vi "Reset.vi"(8 "error in (no error)":errorcluster, 10 "Reset":bool, 11 "ControlState in":T1 {"ChainMask" format="0x%02x"}) -> (0 "error out":errorcluster, 3 "ControlState out":T1 {"ChainMask" format="0x%02x"})   [LabVIEW 2018, in "ArduinoSerialBling.lvlib"]
uses:
  ArduinoSerialBling.lvlib
  ControlState.ctl
  ConnectionType.ctl
  UdpConnection.ctl
  ChainState.ctl
  TransmissionType.ctl
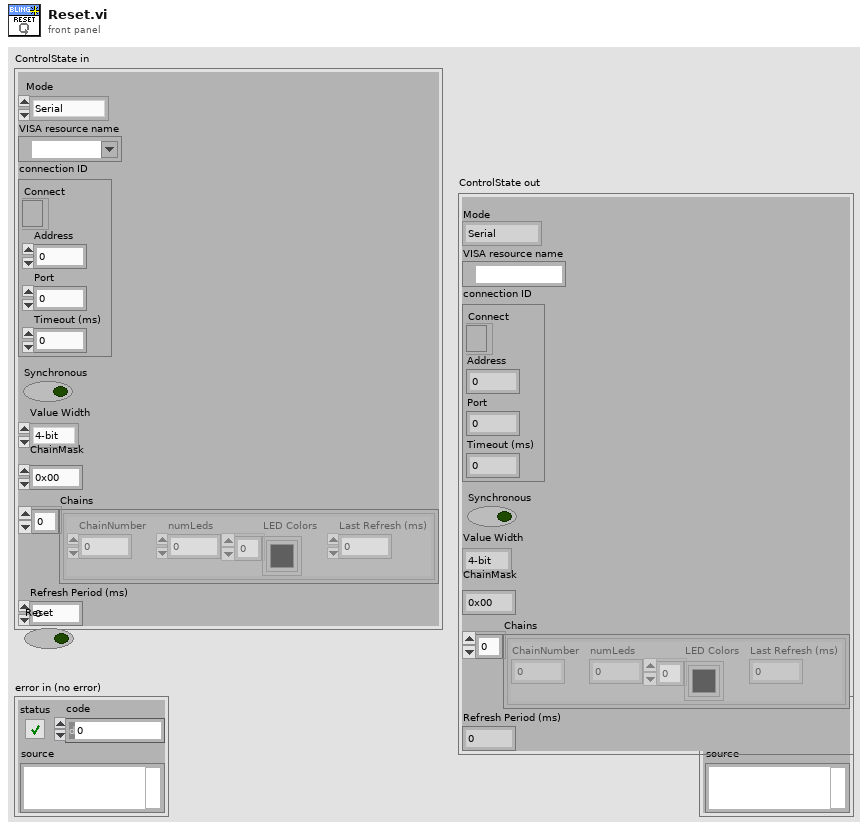
[diagram p1: front panel]
types:
  T1 = typedef "ArduinoSerialBling.lvlib/ControlState.ctl" = cluster{"Mode":T2, "VISA resource name":refnum<visa-resource-name>, "connection ID":T3, "Synchronous":bool, "Value Width":enum16{"4-bit", "8-bit"}, "ChainMask":u8, "Chains":T4[], "Refresh Period (ms)":u32}
  T2 = typedef "ConnectionType.ctl" = enum16{"Serial", "Ethernet", "Offline"}
  T3 = typedef "UdpConnection.ctl" = cluster{"Connect":refnum<k16>, "Address":u32, "Port":u16, "Timeout (ms)":i32}
  T4 = typedef "ArduinoSerialBling.lvlib/ChainState.ctl" = cluster{"ChainNumber":u8, "numLeds":u8, "LED Colors":u32[], "Last Refresh (ms)":u32}
  T5 = typedef "ArduinoSerialBling.lvlib/TransmissionType.ctl" = enum16{"Follow Global", "Asynchronous", "Synchronous"}
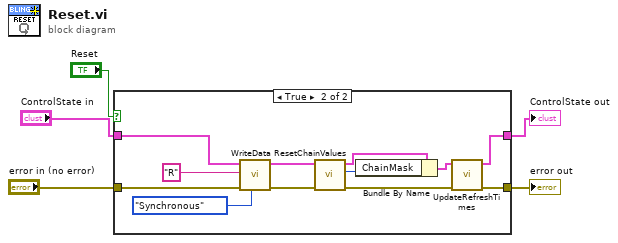
[diagram p0: block diagram]
diagram:
  n1 = case shown="True" "Reset" {
    tunnel: [w7 w9] -> w4
    tunnel: "error in (no error)" -> [w7 w17]
    tunnel: "ControlState in" -> [w6 w18]
    tunnel: [w6 w8] -> w1
    frame False {
    }
    frame True {
      n2 = call "WriteData.vi"("TransmissionType"=TransmissionType."Synchronous", "error in (no error)"=w17, "Command"="R" ("write buffer"), "ControlState in"=w18) -> ("error out"=w15:errorcluster, "ControlState out"=w13:T1)  [unwired: 4 in, 2 out]
      n3 = call "ResetChainValues.vi"("error in (no error)"=w15, "ControlState in"=w13) -> ("error out"=w14:errorcluster, "ChainMask"=w12:u8, "ControlState out"=w10:T1)  [unwired: 7 in]
      n4 = Bundle By Name(cluster=w10, "ChainMask"=w12) -> (w11:T1)
      n5 = call "UpdateRefreshTimes.vi"("error in (no error)"=w14, "ControlState in"=w11) -> ("error out"=w9:errorcluster, "ControlState out"=w8:T1)  [unwired: 8 in]
    }
  }
  "error out" <- w4
  "ControlState out" <- w1
